vi "Edit trap cluster.vi"(2 "Coordinate mapping \n(IMAQ to SLM)":T1={"cZ"=1.0, "cY"=0.15130024, "cX"=0.15130024, "sZ"=0.0, "sY"=-89.04019, "sX"=-116.27423}, 3 "trap cluster in":T2={"X (IMAQ)"=[451.25, 662.75, 874.25, 1085.75], "Y (IMAQ)"=[852.875, 852.875, 852.875, 852.875], "Z"=[0.0, 0.0, 0.0, 0.0], "I"=[70.0, 10.0, 10.0, 10.0], "Trap number"=[0, 1, 2, 3], "ROI number"=[0, 1, 2, 3], "Number of traps"=4, "Group"=[FALSE, FALSE, FALSE, FALSE]}) -> (0 "SubVI closed":bool=TRUE, 1 "Trap cluster out":T2={"X (IMAQ)"=[451.25, 662.75, 874.25, 1085.75], "Y (IMAQ)"=[852.875, 852.875, 852.875, 852.875], "Z"=[0.0, 0.0, 0.0, 0.0], "I"=[70.0, 10.0, 10.0, 10.0], "Trap number"=[0, 1, 2, 3], "ROI number"=[0, 1, 2, 3], "Number of traps"=4, "Group"=[FALSE, FALSE, FALSE, FALSE]})   [LabVIEW 2012]
uses:
  Trap cluster.ctl
panel:
  in  "Use SLM \ncoordinate system":bool=TRUE
  in  "Delete":bool[](array[boolean])=[FALSE, FALSE, FALSE, FALSE]
  in  "Close":bool
  out "ROI number":i32[](array[numeric])=[0, 1, 2, 3]
  in  "Group":bool[](array[boolean])=[FALSE, FALSE, FALSE, FALSE]
  out "Trap#":i32[](array[numeric])=[0, 1, 2, 3]
  in  "I":sgl[](array[numeric])=[10.0, 10.0, 10.0, 10.0]
  in  "Z":sgl[](array[numeric])=[0.0, 0.0, 0.0, 0.0]
  in  "Y":sgl[](array[numeric])=[40.0, 40.0, 40.0, 40.0]
  in  "X":sgl[](array[numeric])=[-48.0, -16.0, 16.0, 48.0]
  in  "Generate grid":bool
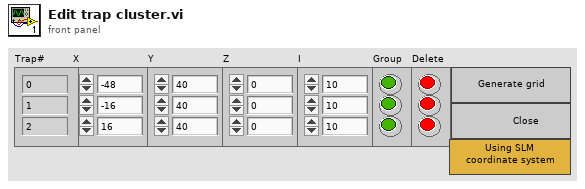
[diagram p1: front panel]
types:
  T1 = cluster{"cZ":sgl, "cY":sgl, "cX":sgl, "sZ":sgl, "sY":sgl, "sX":sgl}
  T2 = typedef "Trap cluster.ctl" = cluster{"X (IMAQ)":sgl[], "Y (IMAQ)":sgl[], "Z":sgl[], "I":sgl[], "Trap number":i32[], "ROI number":i32[], "Number of traps":i32, "Group":bool[]}
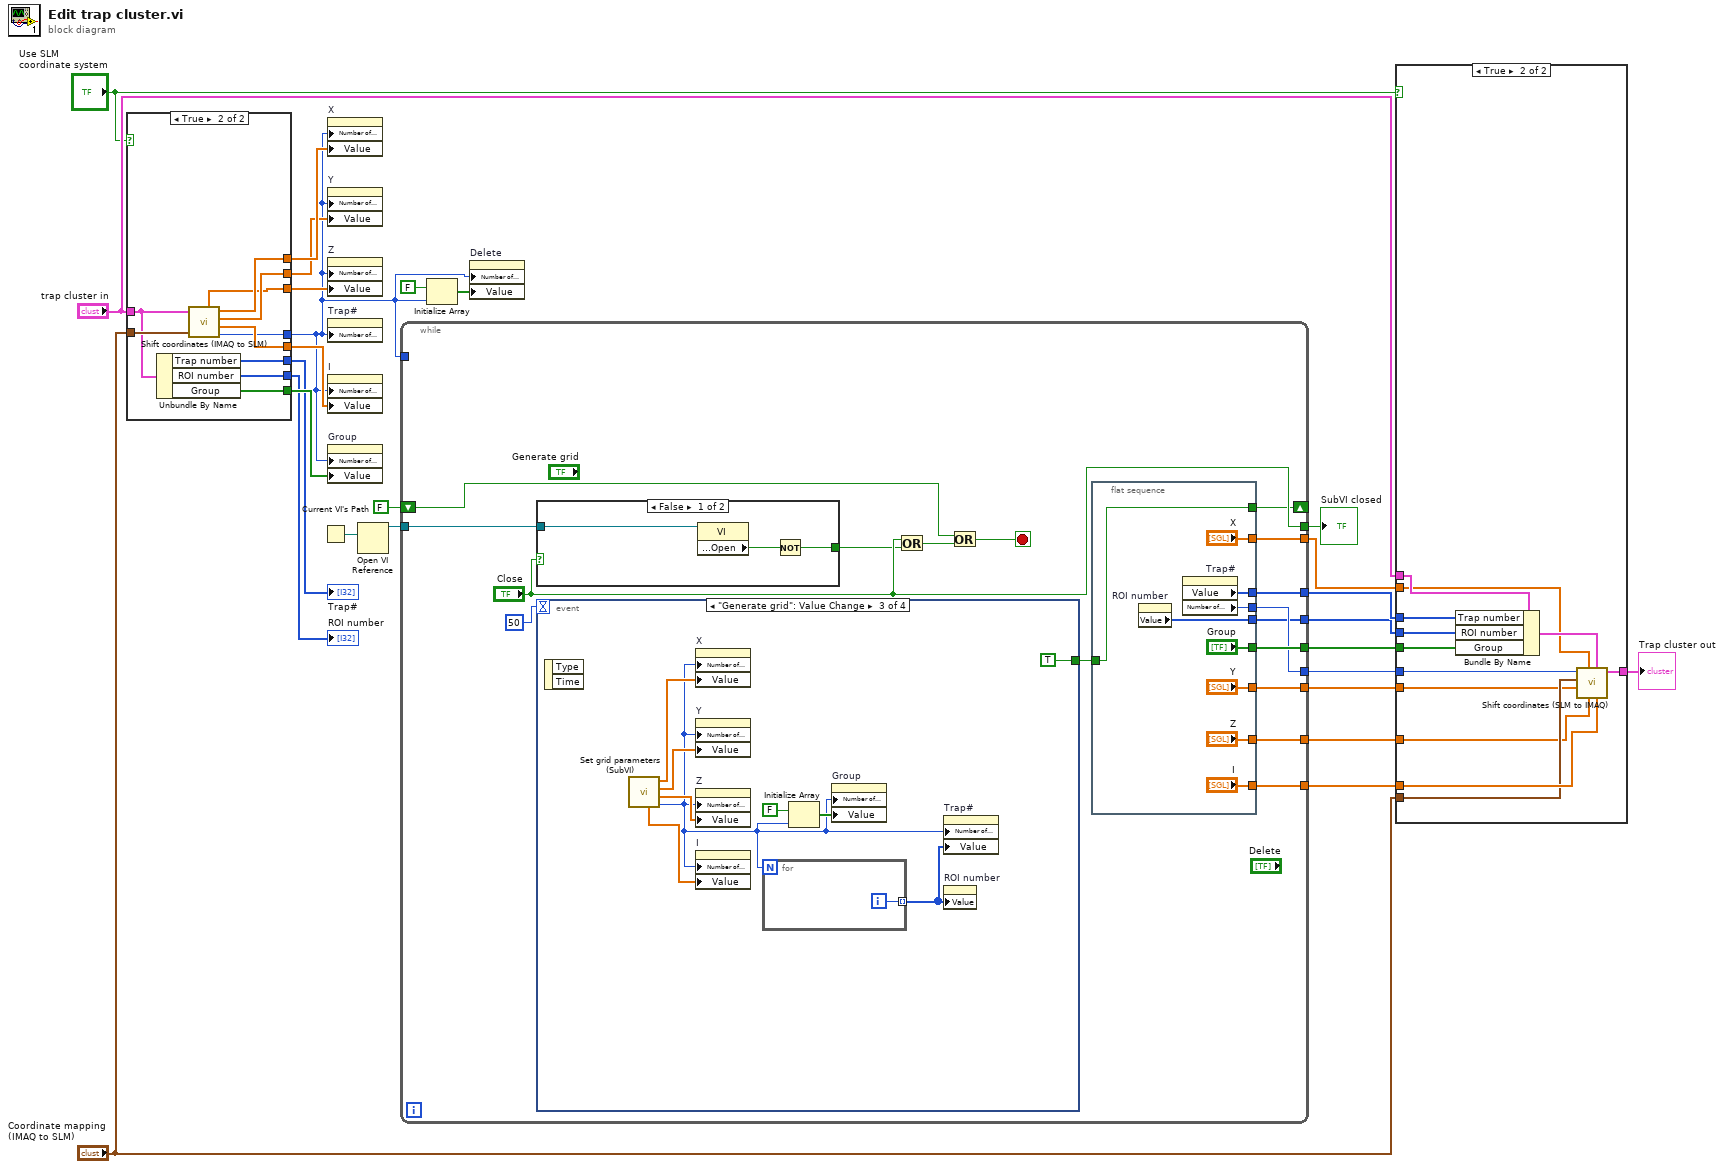
[diagram p0: block diagram]
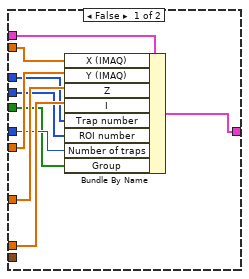
[diagram p2: hidden frame]
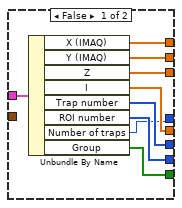
[diagram p3: hidden frame]
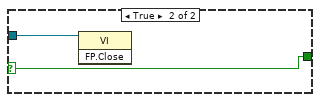
[diagram p4: hidden frame]
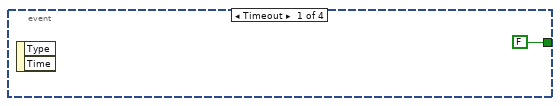
[diagram p5: hidden frame]
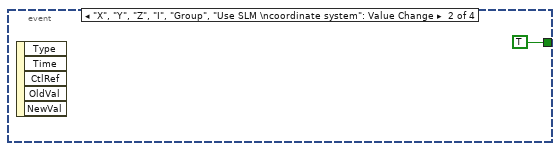
[diagram p6: hidden frame]
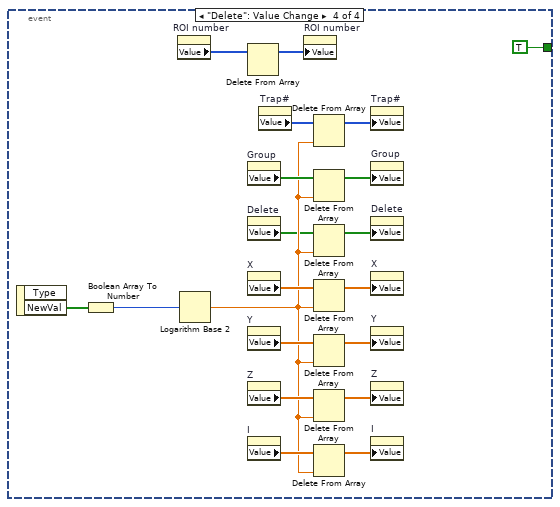
[diagram p7: hidden frame]
diagram:
  n1 = case shown="True" "Use SLM \ncoordinate system" {
    tunnel: [w35 w41] -> w26
    tunnel: [w34 w44] -> w25
    tunnel: [w33 w43] -> w24
    tunnel: [w32 w42] -> w23
    tunnel: [w31 w36] -> w22
    tunnel: [w30 w38] -> w20
    tunnel: [w29 w37] -> w19
    tunnel: "trap cluster in" -> [w28 w39]
    tunnel: [w27 w40] -> w11
    tunnel: "Coordinate mapping \n(IMAQ to SLM)" -> [_ w45]
    frame False {
      n2 = Unbundle By Name(w28) -> ("X (IMAQ)"=w34:sgl[], "Y (IMAQ)"=w33:sgl[], "Z"=w35:sgl[], "I"=w32:sgl[], "Trap number"=w30:i32[], "ROI number"=w29:i32[], "Number of traps"=w27:i32, "Group"=w31:bool[])
    }
    frame True {
      n3 = Unbundle By Name(w39) -> ("Trap number"=w38:i32[], "ROI number"=w37:i32[], "Group"=w36:bool[])
      n4 = call "Shift coordinates (IMAQ to SLM).vi"("Trap cluster"=w39, "Coordinate mapping \n(IMAQ to SLM)"=w45) -> ("X (SLM)"=w44:sgl[], "Y (SLM)"=w43:sgl[], "Intensities"=w42:sgl[], "Number of traps"=w40:i32, "Z (SLM)"=w41:sgl[])  [unwired: 1 in]
    }
  }
  "Trap#" <- w20
  "ROI number" <- w19
  n5 = Current VI's Path() -> (path=w2:path)
  n6 = property on="X" class="Arr (strict)"("Number of Rows"=w11, "Value"=w25) -> ()  [unwired: 2 in, 2 out]
  n7 = property on="Y" class="Arr (strict)"("Number of Rows"=w11, "Value"=w24) -> ()  [unwired: 2 in, 2 out]
  n8 = property on="Z" class="Arr (strict)"("Number of Rows"=w11, "Value"=w26) -> ()  [unwired: 2 in, 2 out]
  n9 = property on="Trap#" class="Arr (strict)"("Number of Rows"=w11) -> ()  [unwired: 2 in, 2 out]
  n10 = property on="I" class="Arr (strict)"("Number of Rows"=w11, "Value"=w23) -> ()  [unwired: 2 in, 2 out]
  n11 = property on="Group" class="Arr (strict)"("Number of Rows"=w11, "Value"=w22) -> ()  [unwired: 2 in, 2 out]
  n12 = Open VI Reference(vi path=w2) -> (vi reference=w1:refnum<vi>)  [unwired: 5 in, 1 out]
  n13 = while {
    tunnel: [w62] -> w10
    tunnel: [w58] -> w6
    tunnel: [w61] -> w5
    tunnel: [w60] -> w8
    tunnel: [w59] -> w21
    tunnel: [w57] -> w18
    tunnel: [w56] -> w9
    tunnel: [w55] -> w17
    shift-right: [w49] -> _
    shift-left: FALSE -> [w53]
    tunnel: ["Close"] -> w14
    tunnel: w11 -> [_]
    tunnel: w1 -> [w48]
    stop <- w52 stop-if-true
    n14 = case shown="False" "Close" {
      selector: "Close" -> [_ w75]
      tunnel: w48 -> [w74 w76]
      tunnel: [w72 w75] -> w46
      frame False {
        n15 = property class="VI"(reference=w74) -> ("Front Panel.Open"=w73:bool)  [unwired: 1 in, 2 out]
        n16 = Not(x=w73) -> (.not. x?=w72:bool)
      }
      frame True {
        n17 = invoke class="VI" method="FP.Close"(reference=w76) -> ()  [unwired: 2 in, 3 out]
      }
    }
    n18 = event shown="[2] \"Generate grid\": Value Change" {
      selector: _ -> [_ _ _ _]
      dyn-events: _ -> [_ _ _ _]
      timeout: u32 50 ("milliseconds to wait") -> [_ _ _ _]
      tunnel: [FALSE TRUE TRUE TRUE] -> w50
      event Timeout {
        n19 = event-data() -> ()  [unwired: 1 in, 2 out]
      }
      event "X", "Y", "Z", "I", "Group", "Use SLM \ncoordinate system": Value Change {
        n20 = event-data() -> ()  [unwired: 1 in, 5 out]
      }
      event "Generate grid": Value Change {
        n21 = event-data() -> ()  [unwired: 1 in, 2 out]
        n22 = call "Set grid parameters (SubVI).vi"() -> ("number of spots"=w81:i32, "Z"=w85:sgl[], "Y"=w86:sgl[], "X"=w87:sgl[], "I"=w84:sgl[])  [unwired: 7 in]
        n23 = property on="X" class="Arr (strict)"("Number of Rows"=w81, "Value"=w87) -> ()  [unwired: 2 in, 2 out]
        n24 = property on="Y" class="Arr (strict)"("Number of Rows"=w81, "Value"=w86) -> ()  [unwired: 2 in, 2 out]
        n25 = property on="Z" class="Arr (strict)"("Number of Rows"=w81, "Value"=w85) -> ()  [unwired: 2 in, 2 out]
        n26 = property on="I" class="Arr (strict)"("Number of Rows"=w81, "Value"=w84) -> ()  [unwired: 2 in, 2 out]
        n27 = for {
          N: w81 -> [_]
          tunnel: [w88] -> w80 mode=indexing
          i -> [w88]
        }
        n28 = Initialize Array(FALSE, w81) -> (w82:bool[])
        n29 = property on="Group" class="Arr (strict)"("Number of Rows"=w81, "Value"=w82) -> ()  [unwired: 2 in, 2 out]
        n30 = property on="Trap#" class="Arr (strict)"("Number of Rows"=w81, "Value"=w80) -> ()  [unwired: 2 in, 2 out]
        n31 = property on="ROI number" class="Arr (strict)"("Value"=w80) -> ()  [unwired: 2 in, 2 out]
      }
      event "Delete": Value Change {
        n32 = event-data() -> ("NewVal"=w108:bool[])  [unwired: 1 in, 1 out]
        n33 = Boolean Array To Number(Boolean array=w108) -> (number=w107:u32)
        n34 = property on="ROI number" class="Arr (strict)"() -> ("Value"=w97:i32[])  [unwired: 2 in, 2 out]
        n35 = Logarithm Base 2(1:w107) -> (0:w99:dbl)
        n36 = Delete From Array(array=w97) -> (array with subset deleted=w89:i32[])  [unwired: 2 in, 1 out]
        n37 = property on="Group" class="Arr (strict)"() -> ("Value"=w100:bool[])  [unwired: 2 in, 2 out]
        n38 = property on="Delete" class="Arr (strict)"() -> ("Value"=w98:bool[])  [unwired: 2 in, 2 out]
        n39 = property on="X" class="Arr (strict)"() -> ("Value"=w105:sgl[])  [unwired: 2 in, 2 out]
        n40 = property on="Y" class="Arr (strict)"() -> ("Value"=w104:sgl[])  [unwired: 2 in, 2 out]
        n41 = property on="Z" class="Arr (strict)"() -> ("Value"=w103:sgl[])  [unwired: 2 in, 2 out]
        n42 = property on="I" class="Arr (strict)"() -> ("Value"=w102:sgl[])  [unwired: 2 in, 2 out]
        n43 = property on="Trap#" class="Arr (strict)"() -> ("Value"=w101:i32[])  [unwired: 2 in, 2 out]
        n44 = property on="ROI number" class="Arr (strict)"("Value"=w89) -> ()  [unwired: 2 in, 2 out]
        n45 = Delete From Array(array=w101, index=w99) -> (array with subset deleted=w92:i32[])  [unwired: 1 in, 1 out]
        n46 = Delete From Array(array=w100, index=w99) -> (array with subset deleted=w91:bool[])  [unwired: 1 in, 1 out]
        n47 = Delete From Array(array=w98, index=w99) -> (array with subset deleted=w90:bool[])  [unwired: 1 in, 1 out]
        n48 = Delete From Array(array=w105, index=w99) -> (array with subset deleted=w96:sgl[])  [unwired: 1 in, 1 out]
        n49 = Delete From Array(array=w104, index=w99) -> (array with subset deleted=w95:sgl[])  [unwired: 1 in, 1 out]
        n50 = Delete From Array(array=w103, index=w99) -> (array with subset deleted=w94:sgl[])  [unwired: 1 in, 1 out]
        n51 = Delete From Array(array=w102, index=w99) -> (array with subset deleted=w93:sgl[])  [unwired: 1 in, 1 out]
        n52 = property on="Trap#" class="Arr (strict)"("Value"=w92) -> ()  [unwired: 2 in, 2 out]
        n53 = property on="Group" class="Arr (strict)"("Value"=w91) -> ()  [unwired: 2 in, 2 out]
        n54 = property on="Delete" class="Arr (strict)"("Value"=w90) -> ()  [unwired: 2 in, 2 out]
        n55 = property on="X" class="Arr (strict)"("Value"=w96) -> ()  [unwired: 2 in, 2 out]
        n56 = property on="Y" class="Arr (strict)"("Value"=w95) -> ()  [unwired: 2 in, 2 out]
        n57 = property on="Z" class="Arr (strict)"("Value"=w94) -> ()  [unwired: 2 in, 2 out]
        n58 = property on="I" class="Arr (strict)"("Value"=w93) -> ()  [unwired: 2 in, 2 out]
      }
    }
    n59 = Or(x="Close", y=w46) -> (x .or. y?=w47:bool)
    n60 = Or(x=w53, y=w47) -> (x .or. y?=w52:bool)
    n61 = flat-sequence {
      tunnel: ["X"] -> w62
      tunnel: ["Z"] -> w61
      tunnel: ["I"] -> w60
      tunnel: ["Group"] -> w59
      tunnel: ["Y"] -> w58
      tunnel: [w66] -> w57
      tunnel: [w65] -> w56
      tunnel: [w64] -> w55
      tunnel: w50 -> [w63]
      tunnel: [w63] -> w49
      frame #0 {
        n62 = property on="ROI number" class="Arr (strict)"() -> ("Value"=w64:i32[])  [unwired: 2 in, 2 out]
        n63 = property on="Trap#" class="Arr (strict)"() -> ("Value"=w66:i32[], "Number of Rows"=w65:u32)  [unwired: 2 in, 2 out]
      }
    }
  }
  "SubVI closed" <- w14
  n64 = Initialize Array(FALSE, w11) -> (w12:bool[])
  n65 = property on="Delete" class="Arr (strict)"("Number of Rows"=w11, "Value"=w12) -> ()  [unwired: 2 in, 2 out]
  n66 = case shown="True" "Use SLM \ncoordinate system" {
    tunnel: w21 -> [w110 w130]
    tunnel: w18 -> [w112 w129]
    tunnel: w17 -> [w113 w128]
    tunnel: "trap cluster in" -> [w118 w127]
    tunnel: w10 -> [w117 w125]
    tunnel: w9 -> [w111 w124]
    tunnel: w8 -> [w114 w123]
    tunnel: "Coordinate mapping \n(IMAQ to SLM)" -> [_ w122]
    tunnel: w6 -> [w116 w121]
    tunnel: w5 -> [w115 w120]
    tunnel: [w109 w119] -> w4
    frame False {
      n67 = Bundle By Name(cluster=w118, "X (IMAQ)"=w117, "Y (IMAQ)"=w116, "Z"=w115, "I"=w114, "Trap number"=w112, "ROI number"=w113, "Number of traps"=w111, "Group"=w110) -> (w109:T2)
    }
    frame True {
      n68 = Bundle By Name(cluster=w127, "Trap number"=w129, "ROI number"=w128, "Group"=w130) -> (w126:T2)
      n69 = call "Shift coordinates (SLM to IMAQ).vi"("I"=w123, "trap cluster in in"=w126, "Z"=w120, "X"=w125, "Y"=w121, "Coordinate mapping \n(IMAQ to SLM)"=w122, "Number of Rows"=w124) -> ("trap cluster in out"=w119:T2)  [unwired: 4 in]
    }
  }
  "Trap cluster out" <- w4
